vi "TagDB Ref to DVR.vi"(4 "TagDB":T1) -> (1 "DVR":refnum<data-value>)   [LabVIEW 2017, in "TagDB.lvlib"]
doc: "Type casts a queue refnum to a message queue refnum."
uses:
  TagDB.lvlib
  Typedef/TagDB.ctl
  Typedef/tagdb-data.ctl
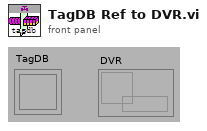
[diagram p1: front panel]
types:
  T1 = typedef "TagDB.lvlib/TagDB.ctl" = refnum<k1>
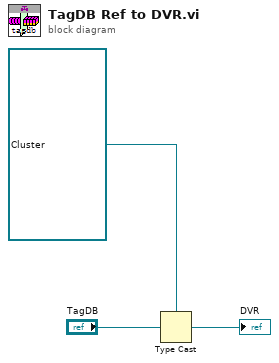
[diagram p0: block diagram]
diagram:
  n1 = Type Cast(type=refnum<data-value> refnum ("DVR"), x="TagDB") -> (*(type *) &x=→"DVR":refnum<data-value>)
